vi "CSTK_QD_MCListbox Designer.vi"(6 "Variant in":variant, 7 "Shift Pressed?":bool, 8 "error in (no error)":errorcluster, 10 "QD Combo Box Ref":refnum<vi>, 11 "QD Launch VI Ref":refnum<vi>) -> (0 "error out":errorcluster, 4 "Variant out":variant)   [LabVIEW 2015]
doc: "打开MCListbox设计器\n\n默认快捷键 - [M]"
uses:
  Library/MCListbox Designer/CSTK_MCListbox_Designer.vi
  Library/MCListbox Designer/CSTK_MCListbox Designer.lvlib
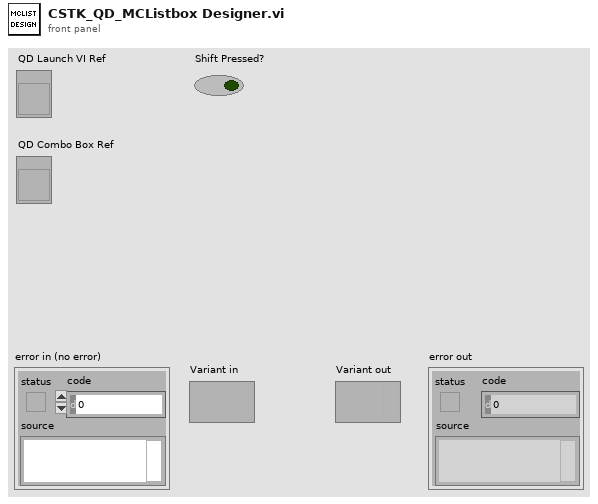
[diagram p1: front panel]
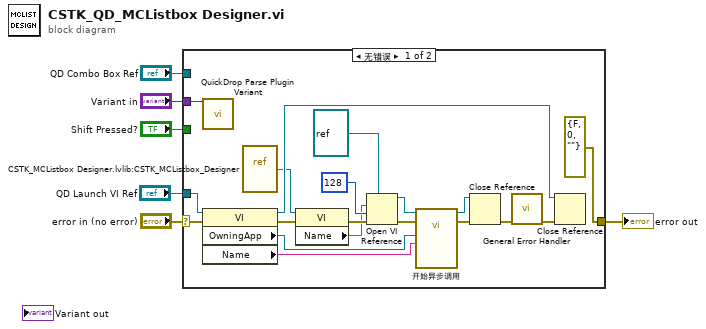
[diagram p0: block diagram]
diagram:
  n1 = case shown="无错误" "error in (no error)" {
    selector: "error in (no error)" -> [w15 w26]
    tunnel: [errorcluster {"status"=FALSE, "code"=0, "source"=""} ("错误常量") w26] -> w5
    tunnel: "QD Launch VI Ref" -> [w16 _]
    tunnel: "Shift Pressed?" -> [_ _]
    tunnel: "QD Combo Box Ref" -> [_ _]
    tunnel: "Variant in" -> [w25 _]
    frame No Error {
      n2 = call <vilib>:"QuickDrop Parse Plugin Variant.vi"("QDKS Variant in"=w25) -> ()  [unwired: 12 in, 3 out]
      n3 = property class="VI"(reference=w16, error in=w15) -> (reference out=w10:refnum<vi>, error out=w12:errorcluster, "OwningApp"=w14:refnum<vi>, "Name"=w13:string)
      n4 = vi-ref "CSTK_MCListbox Designer.lvlib:CSTK_MCListbox_Designer.vi"() -> (w7:refnum<vi>)
      n5 = property class="VI"(reference=w7, error in=w12) -> (error out=w22:errorcluster, "Name"=w17:string)  [unwired: 1 out]
      n6 = Open VI Reference(type specifier VI Refnum (for type only)=refnum<vi> refnum ("类型说明符VI引用句柄（仅用于类型）"), vi path=w17, options=128 ("选项"), error in (no error)=w22) -> (vi reference=w18:refnum<vi>, error out=w19:errorcluster)  [unwired: 2 in]
      n7 = call-by-ref "开始异步调用"(reference=w18, error in=w19, "应用程序:菜单启动:VI"=w13, "应用程序引用（本地）"=w14) -> (reference out=w20:refnum<vi>, error out=w21:errorcluster)  [unwired: 10 in]
      n8 = Close Reference(reference=w20, error in (no error)=w21) -> (error out=w11:errorcluster)
      n9 = call <vilib>:"General Error Handler.vi"("error in (no error)"=w11) -> ("error out"=w9:errorcluster)  [unwired: 10 in, 4 out]
      n10 = Close Reference(reference=w10, error in (no error)=w9) -> ()  [unwired: 1 out]
    }
    frame Error {
    }
  }
  "error out" <- w5
